vi "_4Fare_degree.vi"() -> ()   [LabVIEW 2018]
panel:
  out "Value_2":dbl
  out "Value_1":dbl
  out "Thermometer(C)":dbl(slide) scale=0.0..100.0
  in  "Temperature(F)":dbl(slide) scale=0.0..200.0
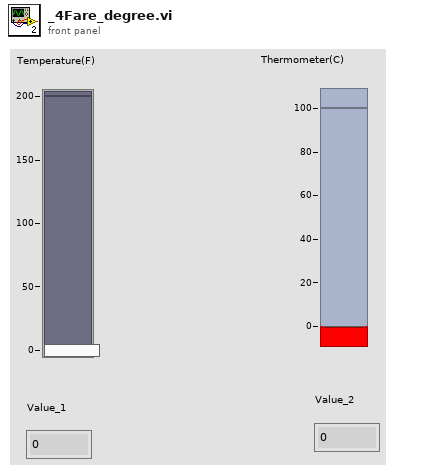
[diagram p1: front panel]
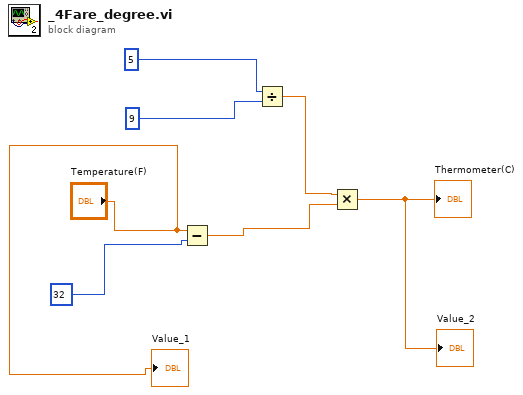
[diagram p0: block diagram]
diagram:
  n1 = Subtract(x="Temperature(F)", y=32) -> (x-y=w3:dbl)
  n2 = Divide(x=5, y=9) -> (x/y=w4:dbl)
  n3 = Multiply(x=w4, y=w3) -> (x*y=→"Thermometer(C)" →"Value_2":dbl)
  "Value_1" <- "Temperature(F)"
